vi "EliminateDuplicates.vi"(11 "Polyline Points in":dbl[][](array[numeric])) -> (3 "Polyline Points out":dbl[][](array[numeric]))   [LabVIEW 2019]
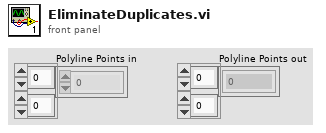
[diagram p1: front panel]
types:
  T1 = cluster{"Polyline Points in[0]":dbl, "Polyline Points in[1]":dbl, "Polyline Points in[2]":dbl, "Polyline Points in[3]":dbl, "Polyline Points in[4]":dbl, "Polyline Points in[5]":dbl, "Polyline Points in[6]":dbl, "Polyline Points in[7]":dbl, "Polyline Points in[8]":dbl}
  T2 = cluster{"Polyline Points in[0]":dbl, "Polyline Points in[1]":dbl, "Polyline Points in[2]":dbl, "Polyline Points in[3]":dbl, "Polyline Points in[4]":dbl, "Polyline Points in[5]":dbl, "Polyline Points in[6]":dbl, "Polyline Points in[7]":dbl, "Polyline Points in[8]":dbl}[]
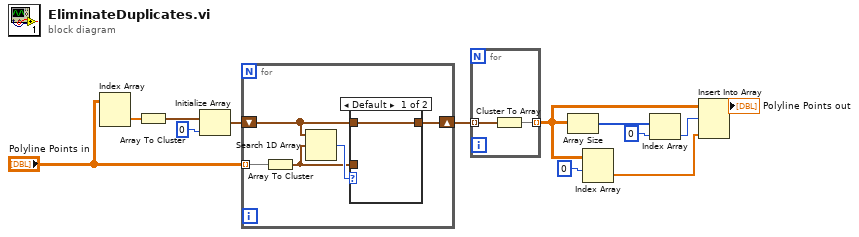
[diagram p0: block diagram]
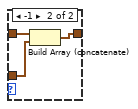
[diagram p2: hidden frame]
diagram:
  n1 = Index Array(array="Polyline Points in") -> (element=w1:dbl[])  [unwired: 2 in]
  n2 = Array To Cluster(array=w1) -> (cluster=w2:T1)
  n3 = Initialize Array(w2, 0 ("Dimension Size")) -> (w4:T2)
  n4 = for {
    tunnel: "Polyline Points in" -> [w17] mode=indexing
    shift-right: [w14] -> w5
    shift-left: w4 -> [w16]
    n5 = Array To Cluster(array=w17) -> (cluster=w15:T1)
    n6 = Search 1D Array(1D array=w16, element=w15) -> (index of element=w18:i32)  [unwired: 1 in]
    n7 = case shown="Default" w18 {
      tunnel: [w19 w22] -> w14
      tunnel: w16 -> [w19 w21]
      tunnel: w15 -> [_ w20]
      frame Default {
      }
      frame -1 {
        n8 = Build Array (concatenate)(w21, w20) -> (w22:T2)
      }
    }
  }
  n9 = for {
    tunnel: w5 -> [w24] mode=indexing
    tunnel: [w23] -> w12 mode=indexing
    n10 = Cluster To Array(cluster=w24) -> (array=w23:dbl[])
  }
  n11 = Array Size(array=w12) -> (size(s)=w9:i32[])
  n12 = Index Array(array=w12, index (row)=0) -> (element=w8:dbl[])  [unwired: 1 in]
  n13 = Index Array(array=w9, index=0) -> (element=w11:i32)
  n14 = Insert Into Array(array=w12, index (row)=w11, new element=w8) -> (→"Polyline Points out":dbl[][])  [unwired: 1 in]
